vi "Pass If Equal 1D Array.vi"(6 "delta (optional)":ext, 8 "error in (no error)":errorcluster, 9 "actual":ext[](array[numeric]), 10 "expected":ext[](array[numeric]), 11 "TestCase in":refnum<class "TestCase.lvclass">) -> (0 "error out":errorcluster, 3 "TestCase out":refnum<class "TestCase.lvclass">)   [LabVIEW 2015, in "VITAC.lvlib"]
uses:
  VITAC.lvlib
  <vilib>/addons/_JKI Toolkits/VI Tester/TestCase.llb/TestCase.lvclass
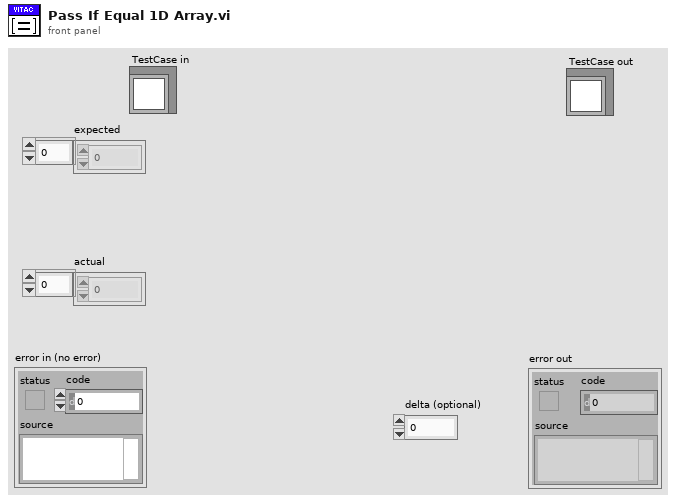
[diagram p1: front panel]
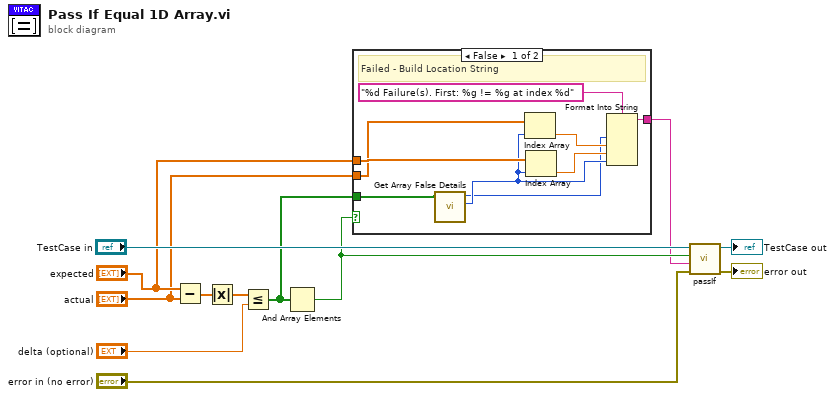
[diagram p0: block diagram]
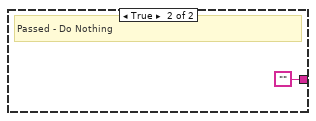
[diagram p2: hidden frame]
diagram:
  n1 = Subtract(x="expected", y="actual") -> (x-y=w8:ext[])
  n2 = Absolute Value(x=w8) -> (abs(x)=w7:ext[])
  n3 = Less Or Equal?(x=w7, y="delta (optional)") -> (x <= y?=w4:bool[])
  n4 = And Array Elements(Boolean array=w4) -> (logical AND=w5:bool)
  n5 = case shown="False" w5 {
    tunnel: w4 -> [w15 _]
    tunnel: "expected" -> [w17 _]
    tunnel: "actual" -> [w16 _]
    tunnel: [w18 ""] -> w1
    frame False {
      # "Failed - Build Location String"
      n6 = call "Get Array False Details.vi"("Array"=w15) -> ("First False"=w14:i32, "Count"=w13:i16)  [unwired: 9 in]
      n7 = Index Array(array=w16, index=w14) -> (element=w20:ext)
      n8 = Index Array(array=w17, index=w14) -> (element=w19:ext)
      n9 = Format Into String(format string="%d Failure(s). First: %g != %g at index %d", w13, w20, w19, w14) -> (resulting string=w18:string)  [unwired: 2 in, 1 out]
    }
    frame True {
      # "Passed - Do Nothing"
    }
  }
  n10 = call-dynamic "passIf.vi"("error in (no error)"="error in (no error)", "message (\"\")"=w1, "pass"=w5, "TestCase in"="TestCase in") -> ("error out"=→"error out":errorcluster, "TestCase out"=→"TestCase out":refnum<class "TestCase.lvclass">)  [unwired: 6 in]
